vi "Initialize.vi"(8 "error in (no error)":errorcluster, 11 "Sync Box in":refnum<class "Sync Box.lvclass">) -> (0 "error out":errorcluster, 3 "Sync Box out":refnum<class "Sync Box.lvclass">)   [LabVIEW 2018, in "Sync Box.lvclass"]
uses:
  Sync Box.lvclass
  C:/Users/observer/Desktop/Sparc4GUI/SPARC4_GUI/Server/Server.lvclass
  Server/Server.lvclass/Server.ctl
  Server/Server.lvclass
  Comm/Stream/Stream.lvclass
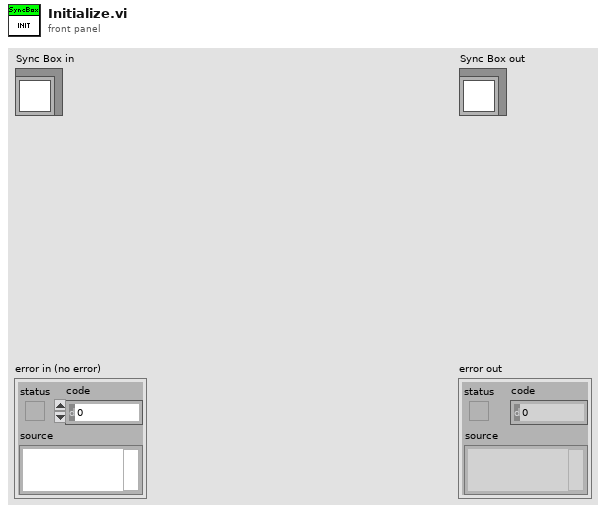
[diagram p1: front panel]
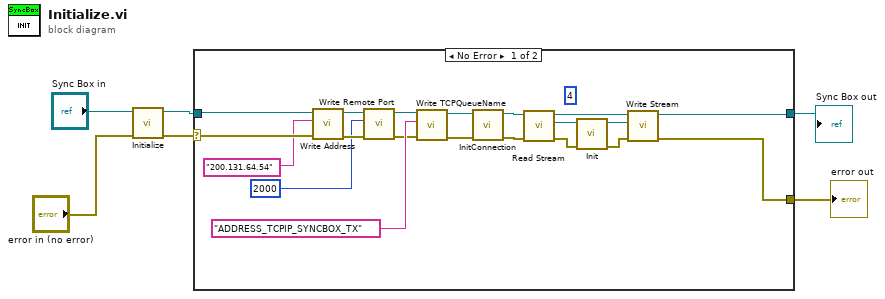
[diagram p0: block diagram]
diagram:
  n1 = call-parent "Initialize.vi"("error in (no error)"="error in (no error)", "Server in"="Sync Box in") -> ("error out"=w1:errorcluster, "Server out"=w4:refnum<class "Sync Box.lvclass">)  [unwired: 8 in]
  n2 = case shown="No Error" w1 {
    selector: w1 -> [w19 w28]
    tunnel: [w7 w28] -> w2
    tunnel: [w8 w27] -> w3
    tunnel: w4 -> [w21 w27]
    frame No Error {
      (unwired) u32 4 ("id")
      n3 = call "Write Address.vi"("error in (no error)"=w19, "Address"="200.131.64.54" ("Address:"), "Server in"=w21) -> ("error out"=w18:errorcluster, "Server out"=w20:refnum<class "Sync Box.lvclass">)  [unwired: 7 in]
      n4 = call "Write Remote Port.vi"("error in (no error)"=w18, "Remote Port"=u32 2000 ("Remote Port:"), "Server in"=w20) -> ("error out"=w11:errorcluster, "Server out"=w12:refnum<class "Sync Box.lvclass">)  [unwired: 7 in]
      n5 = call-dynamic "Write TCPQueueName.vi"("error in (no error)"=w11, "TCPQueueName"="ADDRESS_TCPIP_SYNCBOX_TX", "Server in"=w12) -> ("error out"=w10:errorcluster, "Server out"=w9:refnum<class "Sync Box.lvclass">)  [unwired: 7 in]
      n6 = call-dynamic "InitConnection.vi"("error in (no error)"=w10, "Sync Box in"=w9) -> ("error out"=w14:errorcluster, "Sync Box out"=w15:refnum<class "Sync Box.lvclass">)  [unwired: 8 in]
      n7 = call-dynamic "Read Stream.vi"("error in (no error)"=w14, "Server in"=w15) -> ("error out"=w25:errorcluster, "Stream.lvclass"=w26:refnum<class "Stream.lvclass">, "Server out"=w22:refnum<class "Sync Box.lvclass">)  [unwired: 7 in]
      n8 = call-dynamic "Init.vi"("error in (no error)"=w25, "Stream in"=w26) -> ("error out"=w23:errorcluster, "Stream out"=w24:refnum<class "Stream.lvclass">)  [unwired: 8 in]
      n9 = call-dynamic "Write Stream.vi"("error in (no error)"=w23, "Stream.lvclass"=w24, "Server in"=w22) -> ("error out"=w7:errorcluster, "Server out"=w8:refnum<class "Sync Box.lvclass">)  [unwired: 7 in]
    }
    frame Error {
    }
  }
  "Sync Box out" <- w3
  "error out" <- w2
